vi "Get FPGA Path.vi"(8 "error in (no error)":errorcluster, 11 "Custom Device Ref":T1 format="%.0x") -> (0 "error out":errorcluster, 3 "Path":path)   [LabVIEW 2011, in "Engine Sim RT.lvlib"]
uses:
  Engine Sim RT.lvlib
  <vilib>/NI Veristand/Custom Device API/Custom Device Item Ref.ctl
  Shared/Engine Simulation Global.vi
  <vilib>/NI Veristand/Custom Device API/Get Item Property (Boolean).vi
  <vilib>/NI Veristand/Custom Device API/Get Item Property (Dependent File).vi
  <vilib>/NI Veristand/Custom Device API/Get Item Property (Path).vi
  <vilib>/NI Veristand/Custom Device API/Custom Device API.lvlib
  Engine Simulation Shared.lvlib
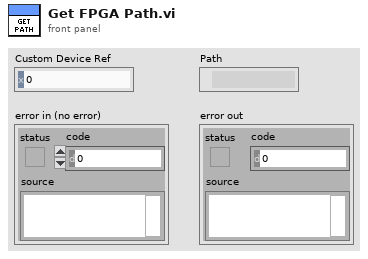
[diagram p1: front panel]
types:
  T1 = typedef "Custom Device API.lvlib/Custom Device Item Ref.ctl" = u64
  T2 = enum32{"invalid OS target", "Mac OS", "Windows 3.1", "Windows 95/NT", "Solaris 1", "Solaris 2", "HP-UX", "PowerMAX", "Linux", "Irix", "Rhapsody", "BeOS", "AIX", "OSF1", "VxWorks", "PharLap", "Carbon", "RTX", "Windows x64", "Linux x64"}
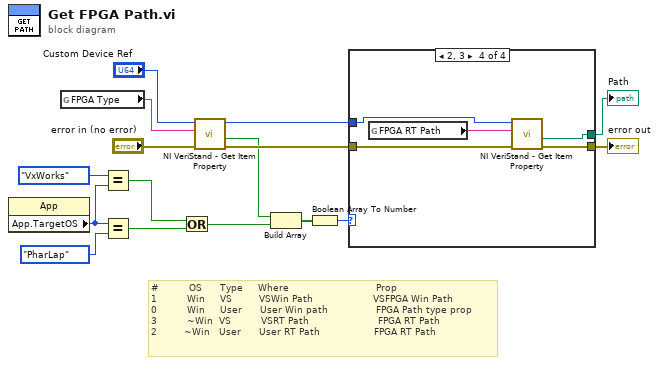
[diagram p0: block diagram]
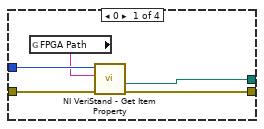
[diagram p2: hidden frame]
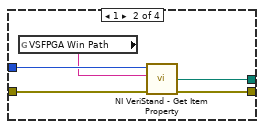
[diagram p3: hidden frame]
diagram:
  # "#          OS      Type     Where                             Prop\n1          Win     VS         VSWin Path                    VSFPGA Win Path\n0          Win     User      User Win path                FPGA Path type prop\n3          ~Win  VS          VSRT Path                       FPGA RT Path\n2         ~Win   User      User RT Path                  FPGA RT Path"
  n1 = property class="App"() -> ("App.TargetOS"=w12:T2)  [unwired: 2 in, 2 out]
  n2 = global read "Engine Simulation Global.vi" "FPGA Type"() -> (w6:string)
  n3 = Equal?(x=T2."VxWorks" ("y"), y=w12) -> (x = y?=w13:bool)
  n4 = Equal?(x=w12, y=T2."PharLap") -> (x = y?=w10:bool)
  n5 = Or(x=w13, y=w10) -> (x .or. y?=w4:bool)
  n6 = call-poly <vilib>:"NI VeriStand - Get Item Property.vi"("error in (no error)"="error in (no error)", "Property Name"=w6, "Item Ref in"="Custom Device Ref") -> ("error out"=w5:errorcluster, "Value"=w1:bool, "Item Ref out"=w8:T1)  [unwired: 5 in, 1 out]
  n7 = Build Array(w1, w4) -> (w3:bool[])
  n8 = Boolean Array To Number(Boolean array=w3) -> (number=w2:u32)
  n9 = case shown="2, 3" w2 {
    tunnel: [w19 w24 w27 w32] -> w16
    tunnel: [w17 w23 _ w31] -> w15
    tunnel: w8 -> [w20 w25 _ w30]
    tunnel: w5 -> [w21 w26 w27 w29]
    frame 0 {
      n10 = global read "Engine Simulation Global.vi" "FPGA Path"() -> (w18:string)
      n11 = call-poly <vilib>:"NI VeriStand - Get Item Property.vi"("error in (no error)"=w21, "Property Name"=w18, "Item Ref in"=w20) -> ("error out"=w19:errorcluster, "Path"=w17:path)  [unwired: 4 in, 3 out]
    }
    frame 1 {
      n12 = global read "Engine Simulation Global.vi" "VSFPGA Win Path"() -> (w22:string)
      n13 = call-poly <vilib>:"NI VeriStand - Get Item Property.vi"("error in (no error)"=w26, "Property Name"=w22, "Item Ref in"=w25) -> ("error out"=w24:errorcluster, "Value"=w23:path)  [unwired: 5 in, 2 out]
    }
    frame Default {
    }
    frame 2, 3 {
      n14 = global read "Engine Simulation Global.vi" "FPGA RT Path"() -> (w28:string)
      n15 = call-poly <vilib>:"NI VeriStand - Get Item Property.vi"("error in (no error)"=w29, "Property Name"=w28, "Item Ref in"=w30) -> ("error out"=w32:errorcluster, "Value"=w31:path)  [unwired: 5 in, 2 out]
    }
  }
  "Path" <- w15
  "error out" <- w16
